vi "ReadCommandData.vi"(8 "error in (no error)":errorcluster, 9 "timeout in ms (-1)":i32, 10 "Messages To Read":u32=2, 11 "Queue in":refnum<queue>) -> (0 "error out":errorcluster, 2 "Data Bytes":u8[](array[numeric]), 3 "Queue in 2":refnum<queue>)   [LabVIEW 2014]
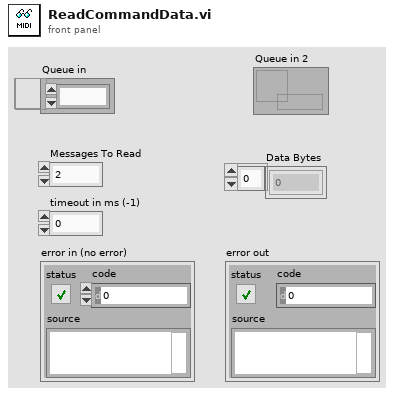
[diagram p1: front panel]
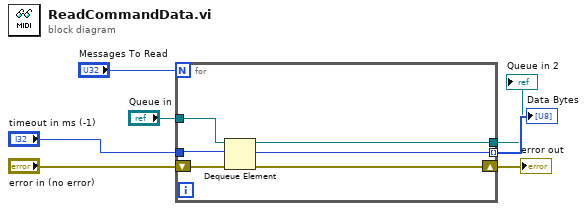
[diagram p0: block diagram]
diagram:
  n1 = for {
    N: "Messages To Read" -> [_]
    shift-right: [w12] -> w5
    shift-left: "error in (no error)" -> [w13]
    tunnel: "Queue in" -> [w10]
    tunnel: [w11] -> w1
    tunnel: "timeout in ms (-1)" -> [w9]
    tunnel: [w8] -> w2 mode=indexing
    n2 = Dequeue Element(queue=w10, timeout in ms (-1)=w9, error in (no error)=w13) -> (queue out=w11:refnum<queue>, element=w8:u8, error out=w12:errorcluster)  [unwired: 1 out]
  }
  "error out" <- w5
  "Data Bytes" <- w2
  "Queue in 2" <- w1
